vi "DMM Wrapper.vi"(7 "Control":T1=enum."Close", 8 "error in":errorcluster, 9 "Alias":string, 10 "Setting":T2={"Resolution (Digits)"=5.5, "Current Source (Amps)"=0.001, "Range (Volts)"=2.0, "Measurement Type"=enum."DC Volts"} {"Range (Volts)" format="%.2p"; "Current Source (Amps)" items=["1uA"=1e-06, "10uA"=1e-05, "100uA"=0.0001, "1mA"=0.001]; "Resolution (Digits)" items=["3 1/2"=3.5, "4 1/2"=4.5, "5 1/2"=5.5, "6 1/2"=6.5, "7 1/2"=7.5]}, 11 "DMM Ref":string="NI_DMM4072_sim") -> (0 "error out":errorcluster, 3 "Measurement":dbl=nan)   [LabVIEW 2021]
uses:
  Controls/DMM Controls.ctl
  Controls/DMM_Data.ctl
  Controls/Measure Type.ctl
  Controls/MUX_Data.ctl
  <vilib>/numeric/Random Number (Range) DBL.vi
  75d991ff-c6d8-42a5-8e8a-1235497a3ef1.vi
  <instrlib>/niDMM/nidmm.llb/niDMM Configure Measurement Digits.vi
  <instrlib>/niSwitch/niSwitch.llb/niSwitch Connect Channels (Multiple).vi
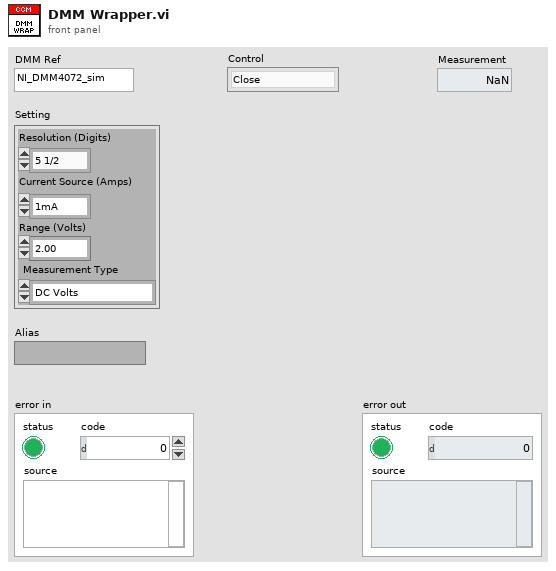
[diagram p1: front panel]
types:
  T1 = typedef "DMM Controls.ctl" = enum16{"Init", "Config", "Read", "Close"}
  T2 = cluster{"Resolution (Digits)":dbl, "Current Source (Amps)":dbl, "Range (Volts)":dbl, "Measurement Type":enum16{"DC Volts", "AC Volts", "DC Current", "AC Current", "2-wire Resistance", "4-wire Resistance", "Diode", "Frequency", "Period", "AC Volts DC Coupled", "Capacitance", "Inductance", "Temperature"}}
  T3 = typedef "Measure Type.ctl" = enum16{"Analog_In", "Analog_Out", "Digital_In", "Digital_Out", "Switch", "NI_DMM"}
  T4 = typedef "MUX_Data.ctl" = cluster{"Alias":string, "Topology":string}
  T5 = cluster{"DMM ref":refnum<k15>, "SW Refs":refnum<k15>[]}
  T6 = typedef "DMM_Data.ctl" = cluster{"Alias":string, "MUX":string, "Route":string}
  T7 = enum16{"DC Volts", "AC Volts", "DC Current", "AC Current", "2-wire Resistance", "4-wire Resistance", "Diode", "Frequency", "Period", "AC Volts DC Coupled", "Capacitance", "Inductance", "Temperature"}
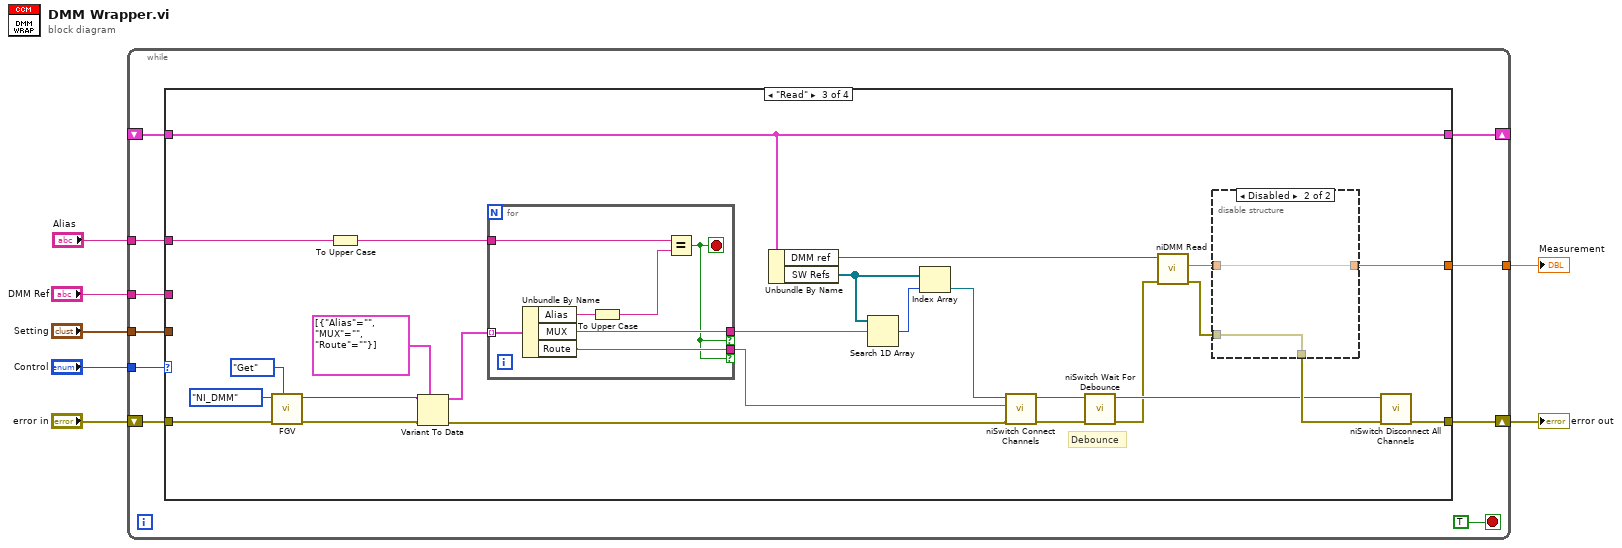
[diagram p0: block diagram]
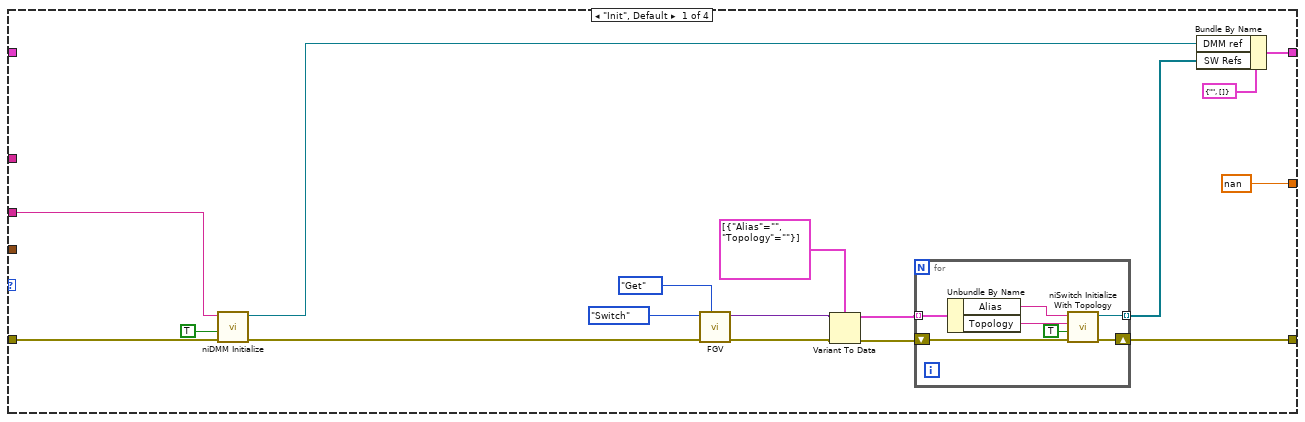
[diagram p2: hidden frame]
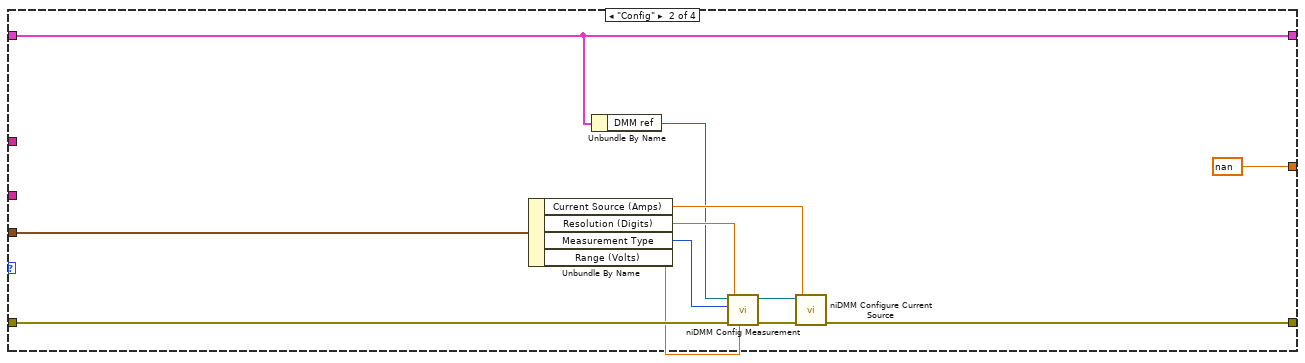
[diagram p3: hidden frame]
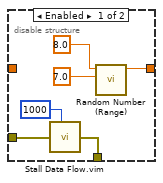
[diagram p4: hidden frame]
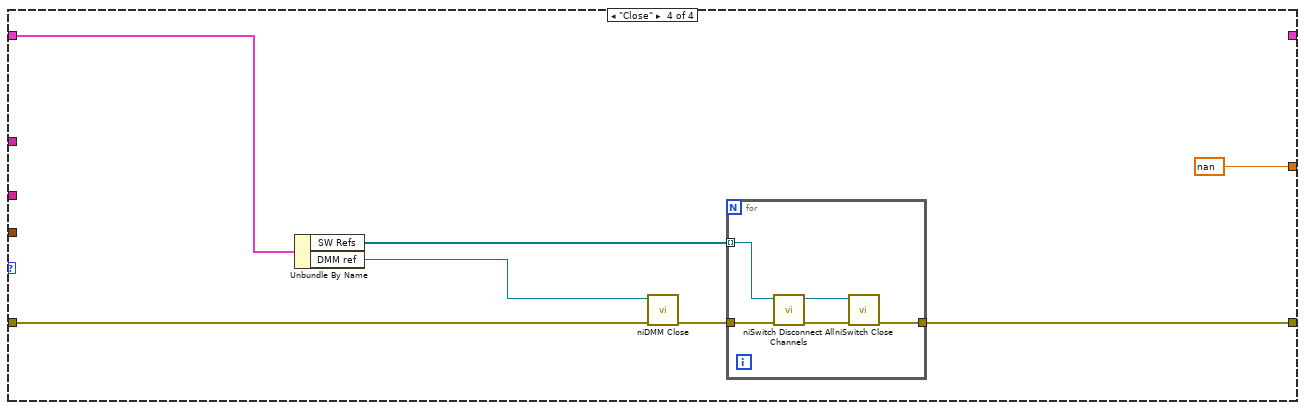
[diagram p5: hidden frame]
diagram:
  n1 = while {
    tunnel: "Setting" -> [w15]
    tunnel: "DMM Ref" -> [w14]
    tunnel: [w13] -> w3
    tunnel: "Control" -> [w12]
    shift-right: [w16] -> w6
    shift-left: "error in" -> [w17]
    shift-right: [w10] -> _
    shift-left: _ -> [w9]
    tunnel: "Alias" -> [w8]
    stop <- TRUE stop-if-true
    n2 = case shown="\"Read\"" w12 {
      tunnel: w17 -> [w19 w52 w61 w96]
      tunnel: [w34 w51 w69 w95] -> w16
      tunnel: [w29 w43 w70 _] -> w10
      tunnel: w9 -> [_ w43 w70 w97]
      tunnel: w15 -> [_ w49 _ _]
      tunnel: w14 -> [w20 _ _ _]
      tunnel: [nan nan w68 nan] -> w13
      tunnel: w8 -> [_ _ w58 _]
      frame "Init", Default {
        n3 = call <instrlib>:"niDMM Initialize.vi"("error in (no error)"=w19, "Reset"=TRUE ("ID Query? (T: Yes)"), "Instrument Descriptor"=w20) -> ("error out"=w27:errorcluster, "instrument handle out"=w31:refnum<k15>)  [unwired: 1 in, 6 out]
        n4 = call "FGV.vi"("Method (Get)"=enum16{"Get", "Set"}."Get", "error in"=w27, "Name"=Measure_Type."Switch") -> ("error out"=w26:errorcluster, "Data out"=w25:variant)  [unwired: 7 in]
        n5 = Variant To Data(error in=w26, type=T4[] [{"Alias"="", "Topology"=""}], Variant=w25) -> (data=w23:T4[], error out=w22:errorcluster)
        n6 = for {
          tunnel: w23 -> [w40] mode=indexing
          tunnel: [w37] -> w30 mode=indexing
          shift-right: [w36] -> w34
          shift-left: w22 -> [w41]
          n7 = Unbundle By Name(w40) -> ("Alias"=w39:string, "Topology"=w38:string)
          n8 = call <instrlib>:"niSwitch Initialize With Topology.vi"("error in (no error)"=w41, "reset device (boolean value)"=TRUE, "topology name"=w38, "resource name"=w39) -> ("error out"=w36:errorcluster, "instrument handle out"=w37:refnum<k15>)  [unwired: 6 in]
        }
        n9 = Bundle By Name(cluster=T5 {"DMM ref"="", "SW Refs"=[]}, "DMM ref"=w31, "SW Refs"=w30) -> (w29:T5)
      }
      frame "Config" {
        n10 = Unbundle By Name(w49) -> ("Current Source (Amps)"=w48:dbl, "Resolution (Digits)"=w47:dbl, "Measurement Type"=w46:T7, "Range (Volts)"=w45:dbl)
        n11 = Unbundle By Name(w43) -> ("DMM ref"=w44:refnum<k15>)
        n12 = call-poly <instrlib>:"niDMM Config Measurement.vi"("Range"=w45, "Resolution in Digits"=w47, "error in (no error)"=w52, "Function"=w46, "instrument handle"=w44) -> ("error out"=w53:errorcluster, "instrument handle out"=w50:refnum<k15>)  [unwired: 5 out]
        n13 = call <instrlib>:"niDMM Configure Current Source.vi"("Current Source"=w48, "error in (no error)"=w53, "instrument handle"=w50) -> ("error out"=w51:errorcluster)  [unwired: 1 in, 7 out]
      }
      frame "Read" {
        # "Debounce"
        n14 = call "FGV.vi"("Method (Get)"=enum16{"Get", "Set"}."Get", "error in"=w61, "Name"=Measure_Type."NI_DMM") -> ("error out"=w65:errorcluster, "Data out"=w64:variant)  [unwired: 7 in]
        n15 = To Upper Case(1:w58) -> (0:w54:string)
        n16 = Variant To Data(error in=w65, type=T6[] [{"Alias"="", "MUX"="", "Route"=""}], Variant=w64) -> (data=w59:T6[], error out=w60:errorcluster)
        n17 = for {
          tunnel: w59 -> [w86] mode=indexing
          tunnel: [w85] -> w57 if=w81
          tunnel: w54 -> [w84]
          tunnel: [w82] -> w56 if=w81
          stop <- w81 stop-if-true
          n18 = Unbundle By Name(w86) -> ("Alias"=w83:string, "MUX"=w85:string, "Route"=w82:string)
          n19 = To Upper Case(1:w83) -> (0:w80:string)
          n20 = Equal?(x=w84, y=w80) -> (x = y?=w81:bool)
        }
        n21 = Unbundle By Name(w70) -> ("DMM ref"=w73:refnum<k15>, "SW Refs"=w75:refnum<k15>[])
        n22 = Search 1D Array(1D array=w75, element=w57) -> (index of element=w74:i32)  [unwired: 1 in]
        n23 = Index Array(array=w75, index=w74) -> (element=w76:refnum<k15>)
        n24 = call-poly <instrlib>:"niSwitch Connect Channels.vi"("error in (no error)"=w60, "connection list"=w56, "instrument handle"=w76) -> ("error out"=w66:errorcluster, "instrument handle out"=w67:refnum<k15>)  [unwired: 7 in]
        n25 = call <instrlib>:"niSwitch Wait For Debounce.vi"("error in (no error)"=w66, "instrument handle"=w67) -> ("error out"=w71:errorcluster, "instrument handle out"=w77:refnum<k15>)  [unwired: 1 in, 7 out]
        n26 = call <instrlib>:"niDMM Read.vi"("error in (no error)"=w71, "instrument handle"=w73) -> ("error out"=w78:errorcluster, "Measurement"=w72:dbl)  [unwired: 1 in, 7 out]
        n27 = disable-structure shown="Disabled" {
          disable-tunnel: w72 -> [_ w94]
          disable-tunnel: [w90 w94] -> w68
          disable-tunnel: w78 -> [w88 w93]
          disable-tunnel: [w87 w93] -> w79
          frame Enabled {
            n28 = call "Stall Data Flow.vim"("value in"=w88, "milliseconds to wait"=u32 1000) -> ("value out"=w87:errorcluster)  [unwired: 1 out]
            n29 = call-poly <vilib>:"Random Number (Range).vi"("lower bound (0)"=7.0, "upper bound (100)"=8.0) -> ("number"=w90:dbl)  [unwired: 9 in]
          }
          frame Disabled {
          }
        }
        n30 = call <instrlib>:"niSwitch Disconnect All Channels.vi"("error in (no error)"=w79, "instrument handle"=w77) -> ("error out"=w69:errorcluster)  [unwired: 8 in, 1 out]
      }
      frame "Close" {
        n31 = Unbundle By Name(w97) -> ("SW Refs"=w100:refnum<k15>[], "DMM ref"=w99:refnum<k15>)
        n32 = call <instrlib>:"niDMM Close.vi"("error in (no error)"=w96, "instrument handle"=w99) -> ("error out"=w98:errorcluster)  [unwired: 9 in]
        n33 = for {
          tunnel: w100 -> [w102] mode=indexing
          tunnel: w98 -> [w103]
          tunnel: [w106] -> w95
          n34 = call <instrlib>:"niSwitch Disconnect All Channels.vi"("error in (no error)"=w103, "instrument handle"=w102) -> ("error out"=w105:errorcluster, "instrument handle out"=w104:refnum<k15>)  [unwired: 8 in]
          n35 = call <instrlib>:"niSwitch Close.vi"("error in (no error)"=w105, "instrument handle"=w104) -> ("error out"=w106:errorcluster)  [unwired: 9 in]
        }
      }
    }
  }
  "error out" <- w6
  "Measurement" <- w3
